vi "4-7.vi"() -> ()   [LabVIEW 2017]
panel:
  out "猜测次数":dbl
  out "随机数":dbl
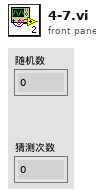
[diagram p1: front panel]
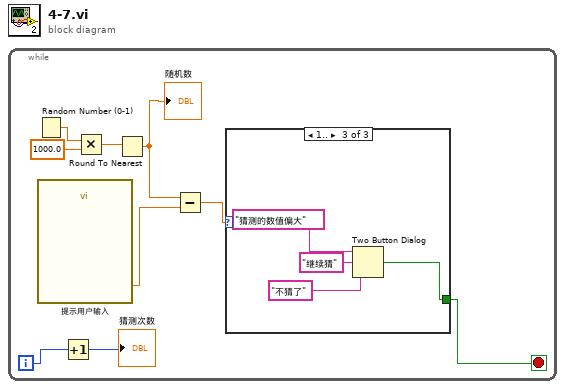
[diagram p0: block diagram]
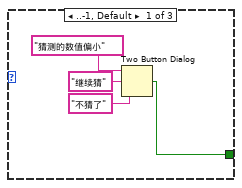
[diagram p2: hidden frame]
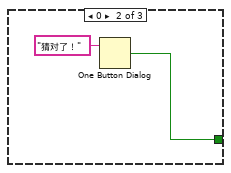
[diagram p3: hidden frame]
diagram:
  n1 = while {
    i -> [w2]
    stop <- w3 stop-if-true
    n2 = Random Number (0-1)() -> (number: 0 to 1=w9:dbl)
    n3 = call "提示用户输入"() -> ("猜测值"=w5:dbl)  [unwired: 17 in, 2 out]
    n4 = Increment(x=w2) -> (x+1=→"猜测次数":i32)
    n5 = Multiply(x=w9, y=1000.0) -> (x*y=w7:dbl)
    n6 = Round To Nearest(number=w7) -> (nearest integer value=w6:dbl)
    "随机数" <- w6
    n7 = Subtract(x=w6, y=w5) -> (x-y=w4:dbl)
    n8 = case shown="1.." w4 {
      tunnel: [w10 w15 w16] -> w3
      frame ..-1, Default {
        n9 = Two Button Dialog(message="猜测的数值偏小" ("消息 2"), 1:"不猜了" ("F按钮名称（“取消”）"), 2:"继续猜" ("T按钮名称（“确定”）")) -> (T button?=w10:bool)
      }
      frame 0 {
        n10 = One Button Dialog(message="猜对了！" ("消息")) -> (true=w15:bool)  [unwired: 1 in]
      }
      frame 1.. {
        n11 = Two Button Dialog(message="猜测的数值偏大" ("消息"), 1:"不猜了" ("F按钮名称（“取消”）"), 2:"继续猜" ("T按钮名称（“确定”）")) -> (T button?=w16:bool)
      }
    }
  }
